vi "Test VI.vi"() -> ()   [LabVIEW 2020]
panel:
  in  "index":i32
  out "element":dbl
  out "size(s)":i32
  in  "Array 2":dbl[](array[slide]) scale=0.0..10.0
  out "Array":dbl[](array[numeric])
  out "Waveform Graph":dbl[](graph)
  in  "stop":bool
  out "Waveform Chart":dbl(graph)
  in  "Convert to C":bool
  out "String 3":string
  in  "String 2":string
  out "Boolean Indicator":bool
  in  "Boolean Control":bool
  out "Floating Point Indicator":dbl
  in  "Floating Point Control":dbl
  out "Integer Indicator":i32
  in  "Integer Control":i32
  out "String":string
  in  "Temperature (F)":dbl(slide) scale=0.0..100.0
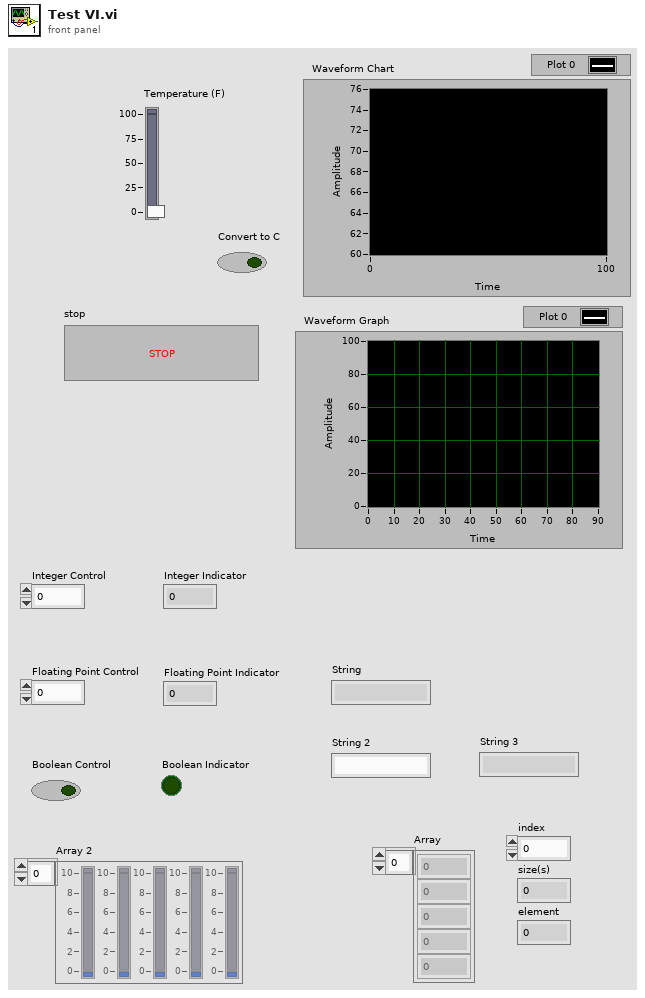
[diagram p1: front panel]
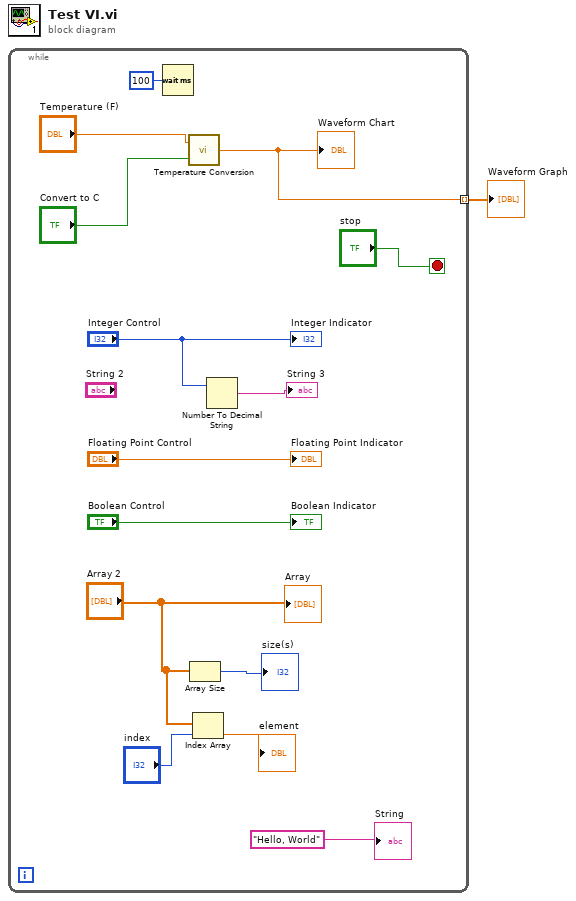
[diagram p0: block diagram]
diagram:
  n1 = while {
    tunnel: [w11] -> w1 mode=indexing
    stop <- "stop" stop-if-true
    n2 = Wait (ms)(milliseconds to wait=u32 100) -> ()  [unwired: 1 out]
    n3 = call "Temperature Conversion.vi"("Convert to C"="Convert to C", "Temperature (F)"="Temperature (F)") -> ("Numeric"=w11:dbl)
    "Waveform Chart" <- w11
    n4 = Array Size(array="Array 2") -> (size(s)=→"size(s)":i32)
    n5 = Index Array(array="Array 2", index="index") -> (element=→"element":dbl)
    n6 = Number To Decimal String(number="Integer Control") -> (decimal integer string=→"String 3":string)  [unwired: 1 in]
    "Integer Indicator" <- "Integer Control"
    "Floating Point Indicator" <- "Floating Point Control"
    "Boolean Indicator" <- "Boolean Control"
    "Array" <- "Array 2"
    "String" <- "Hello, World"
  }
  "Waveform Graph" <- w1
